vi "FolderMon callback changes.vi"(4 "error in (no error)":errorcluster, 6 "Changes":T2, 7 "Callback VI Name (Empty)":string) -> (0 "error out":errorcluster)   [LabVIEW 2011]
uses:
  FolderMon changes.ctl
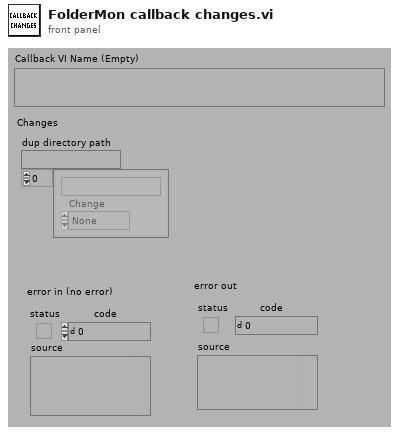
[diagram p1: front panel]
types:
  T1 = typedef "FolderMon changes.ctl" = enum16{"None", "First", "New", "Properties", "Deleted"}
  T2 = cluster{"dup directory path":path, cluster{string, "Change":T1}[]}
  T3 = enum32{"invalid app kind", "Development System", "Run Time System", "Student Edition", "Embedded LabVIEW", "Evaluation", "Custom"}
  T4 = typedef "Rendezvous RefNum" = refnum<k1>
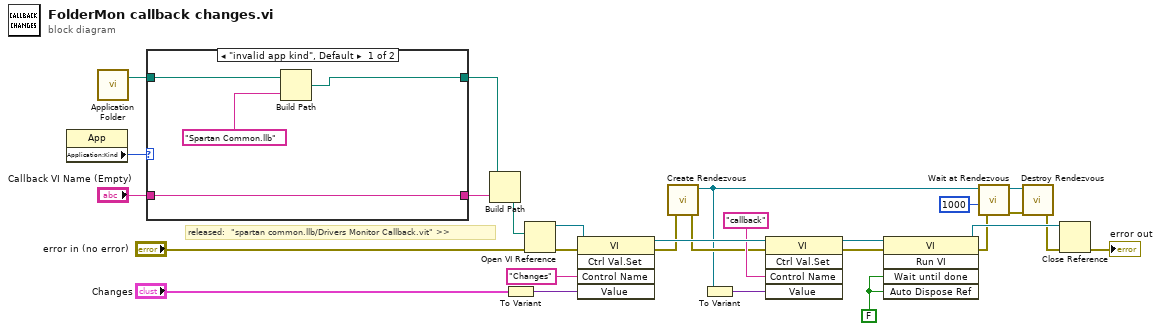
[diagram p0: block diagram]
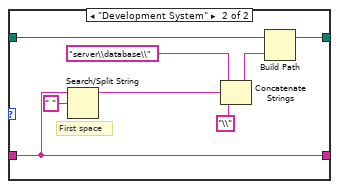
[diagram p2: hidden frame]
diagram:
  w20 = FALSE
  # "released:  \"spartan common.llb/Drivers Monitor Callback.vit\" >>"
  n1 = property class="App"() -> ("Application:Kind"=w5:T3)  [unwired: 2 in, 2 out]
  n2 = call "Application Folder.vi"() -> ("Application Folder"=w4:path)  [unwired: 3 in]
  n3 = case shown="\"invalid app kind\", Default" w5 {
    tunnel: [w30 w39] -> w3
    tunnel: w4 -> [w31 w40]
    tunnel: "Callback VI Name (Empty)" -> [w32 w33]
    tunnel: [w32 w33] -> w1
    frame "invalid app kind", Default {
      n4 = Build Path(base path=w31, name or relative path="Spartan Common.llb") -> (appended path=w30:path)
    }
    frame "Development System" {
      # "First space"
      n5 = Search/Split String(string=w33, search string/char (-)=" ") -> (substring before match=w35:string)  [unwired: 3 out]
      n6 = Concatenate Strings("server\\database\\", w35, "\\") -> (w36:string)
      n7 = Build Path(base path=w40, name or relative path=w36) -> (appended path=w39:path)
    }
  }
  n8 = Build Path(base path=w3, name or relative path=w1) -> (appended path=w6:path)
  n9 = To Variant(anything="Changes") -> (Variant=w21:variant)
  n10 = Open VI Reference(vi path=w6, error in (no error)="error in (no error)") -> (vi reference=w25:refnum<vi>, error out=w24:errorcluster)  [unwired: 4 out]
  n11 = invoke class="VI" method="Ctrl Val.Set"(reference=w25, error in=w24, "Control Name"="Changes", "Value"=w21) -> (reference out=w17:refnum<vi>, error out=w14:errorcluster)  [unwired: 1 in, 3 out]
  n12 = call <vilib>:"Create Rendezvous.vi"("error in (no error)"=w14) -> ("error out"=w13:errorcluster, "rendezvous"=w12:T4)  [unwired: 1 in, 4 out]
  n13 = To Variant(anything=w12) -> (Variant=w19:variant)
  n14 = invoke class="VI" method="Ctrl Val.Set"(reference=w17, error in=w13, "Control Name"="callback", "Value"=w19) -> (reference out=w16:refnum<vi>, error out=w18:errorcluster)  [unwired: 1 in, 3 out]
  n15 = invoke class="VI" method="Run VI"(reference=w16, error in=w18, "Wait until done"=w20, "Auto Dispose Ref"=w20) -> (reference out=w22:refnum<vi>, error out=w8:errorcluster)  [unwired: 1 in, 3 out]
  n16 = call <vilib>:"Wait at Rendezvous.vi"("error in (no error)"=w8, "ms timeout (-1)"=1000, "rendezvous"=w12) -> ("error out"=w10:errorcluster, "rendezvous out"=w9:T4)  [unwired: 3 out]
  n17 = call <vilib>:"Destroy Rendezvous.vi"("error in (no error)"=w10, "rendezvous"=w9) -> ("error out"=w7:errorcluster)  [unwired: 5 out]
  n18 = Close Reference(reference=w22, error in (no error)=w7) -> (error out=→"error out":errorcluster)
